vi "mlink_pwm_write.vi"(4 "channel B":sgl, 6 "channel A":sgl, 7 "PWM module":enum8{"None", "PWM1", "PWM2", "PWM3"}(ring)=enum."PWM1", 8 "error in (no error)":errorcluster, 11 "connection ID":i32=-1) -> (0 "error out":errorcluster, 3 "connection ID out":i32)   [LabVIEW 2009, in "MicroDAQ.lvlib" / "mlink.lvlib"]
doc: "This function sets PWM waveform duty for A and B channels for selected PWM module. PWM module has to be initiated with mlink_pwm_init() function call."
uses:
  <instrlib>/MicroDAQ/Mlink library wraper/mlink.lvlib
  <instrlib>/MicroDAQ/MLink32.dll
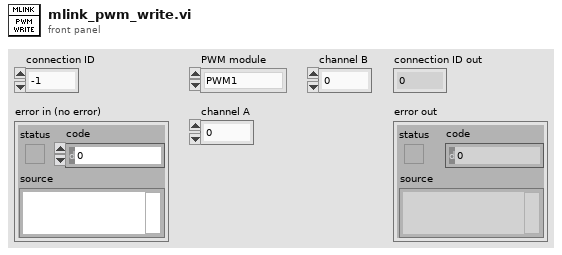
[diagram p1: front panel]
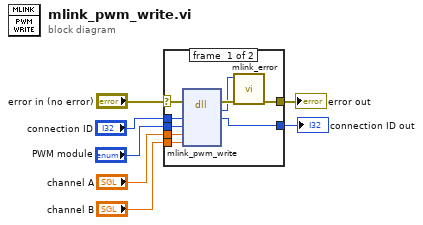
[diagram p0: block diagram]
diagram:
  n1 = case shown="No Error" "error in (no error)" {
    selector: "error in (no error)" -> [w12 w18]
    tunnel: "connection ID" -> [w16 w17]
    tunnel: [w15 w17] -> w6
    tunnel: "channel A" -> [w14 _]
    tunnel: "channel B" -> [w13 _]
    tunnel: [w11 w18] -> w2
    tunnel: "PWM module" -> [w8 _]
    frame #0 {
      n2 = dll-call lib="C:/Program Files (x86)/National Instruments/LabVIEW 2009/instr.lib/MicroDAQ/MLink32.dll" fn="mlink_pwm_write"(error in=w12, "connection ID"=w16, "module"=w8, "channel A"=w14, "channel B"=w13) -> (error out=w10:errorcluster, "return type"=w9:i32, "connection ID"=w15:i32)  [unwired: 5 in, 1 out]
      n3 = call <instrlib>:"mlink_error.vi"("error in (no error)"=w10, "error code"=w9) -> ("error out"=w11:errorcluster)  [unwired: 9 in]
    }
    frame #1 {
    }
  }
  "connection ID out" <- w6
  "error out" <- w2
